vi "get_standardVisitor.vi"(8 "error in (no error)":errorcluster, 11 "HGF_Agent in":refnum<class "MoAgSy_AgentBase.lvclass">) -> (0 "error out":errorcluster, 2 "standard Visitor":T1, 3 "HGF_Agent out":refnum<class "MoAgSy_AgentBase.lvclass">)   [LabVIEW 2009, in "MoAgSy_Base.lvlib" / "MoAgSy_AgentBase.lvclass"]
uses:
  MoAgSy_AgentBase.lvclass
  Visitors/MoAgSy_Visitor/MoAgSy_Visitor.lvclass
  MoAgSy_AgentBase.lvclass/MoAgSy_AgentBase.ctl
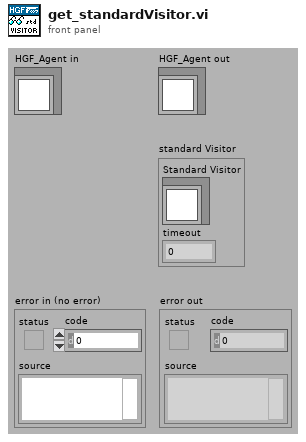
[diagram p1: front panel]
types:
  T1 = cluster{"Standard Visitor":refnum<class "MoAgSy_Visitor.lvclass">, "timeout":dbl}
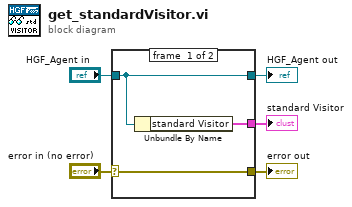
[diagram p0: block diagram]
diagram:
  n1 = case shown="No Error" "error in (no error)" {
    selector: "error in (no error)" -> [w8 w9]
    tunnel: [w8 w9] -> w4
    tunnel: [w7 w10] -> w2
    tunnel: "HGF_Agent in" -> [w7 w10]
    tunnel: [w6 _] -> w1
    frame #0 {
      n2 = Unbundle By Name(w7) -> ("standard Visitor"=w6:T1)
    }
    frame #1 {
    }
  }
  "error out" <- w4
  "HGF_Agent out" <- w2
  "standard Visitor" <- w1
